vi "Get Config File Path.vi"(8 "error in (no error)":errorcluster) -> (0 "error out":errorcluster, 3 "appended path":path)   [LabVIEW 2017, in "Settings.lvclass"]
uses:
  Settings.lvclass
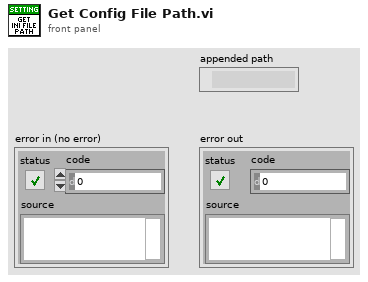
[diagram p1: front panel]
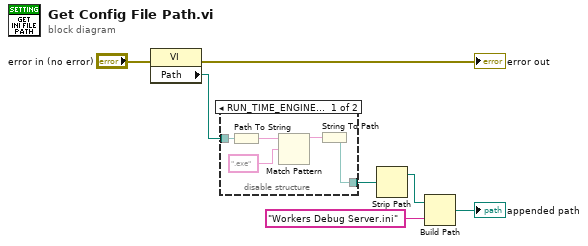
[diagram p0: block diagram]
diagram:
  n1 = property class="VI"(error in="error in (no error)") -> (error out=→"error out":errorcluster, "Path"=w1:path)  [unwired: 1 in, 1 out]
  n2 = disable-structure shown="RUN_TIME_ENGINE==True" {
    disable-tunnel: [w8 w13] -> w6
    disable-tunnel: w1 -> [w11 w13]
    frame condition #0 {
      n3 = Path To String(path=w11) -> (string=w10:string)
      n4 = Match Pattern(string=w10, regular expression=".exe") -> (before substring=w12:string)  [unwired: 1 in, 3 out]
      n5 = String To Path(string=w12) -> (path=w8:path)
    }
    frame condition #1 (active) {
    }
  }
  n6 = Strip Path(path=w6) -> (stripped path=w4:path)  [unwired: 1 out]
  n7 = Build Path(base path=w4, name or relative path="Workers Debug Server.ini") -> (appended path=→"appended path":path)
